vi "Read writeString.vi"(11 "SerialSimulator in":refnum<class "SerialSimulator.lvclass">) -> (2 "writeString":string, 3 "SerialSimulator out":refnum<class "SerialSimulator.lvclass">)   [LabVIEW 2015, in "SerialProtocols.lvlib" / "SerialSimulator.lvclass"]
uses:
  <userlib>/Common/SerialProtocols/SerialProtocol/SerialSimulator/SerialSimulator.lvclass
  <userlib>/Common/SerialProtocols/SerialProtocol/SerialSimulator/SerialSimulator.lvclass/SerialSimulator.ctl
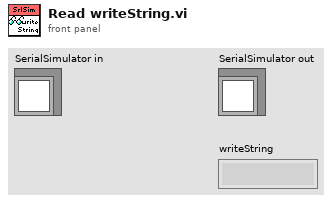
[diagram p1: front panel]
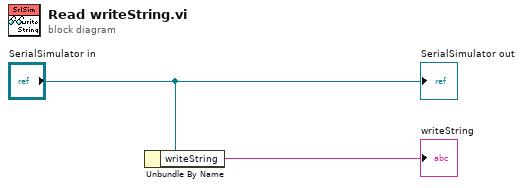
[diagram p0: block diagram]
diagram:
  n1 = Unbundle By Name("SerialSimulator in") -> ("writeString"=→"writeString":string)
  "SerialSimulator out" <- "SerialSimulator in"
